vi "Check Loop Error.vi"(6 "Exit on Error? (F)":bool, 7 "Loop Name":string, 8 "Ignore Errors":i32[](array[numeric]), 9 "error to process":errorcluster, 10 "Database":refnum<queue>, 11 "Message Queue":refnum<queue>) -> (2 "Error?":bool, 3 "dup Message Queue":refnum<queue>)   [LabVIEW 2026]
doc: "Check the 'error to process' to see if its code value matches any of the values in the 'Ignore Errors' array. If so, do nothing. If not, send an \"Error\" message containing the error data to the Message Handling Loop for further processing. If the \"Exit on Error?\" input is TRUE, send an \"Exit\" message to the Message Handling Loop instead."
uses:
  Message Queue/Message Cluster.ctl
  controls/Error_Payload.ctl
  Message Queue/Enqueue Message (Single).vi
  Message Queue/Message Queue.lvlib
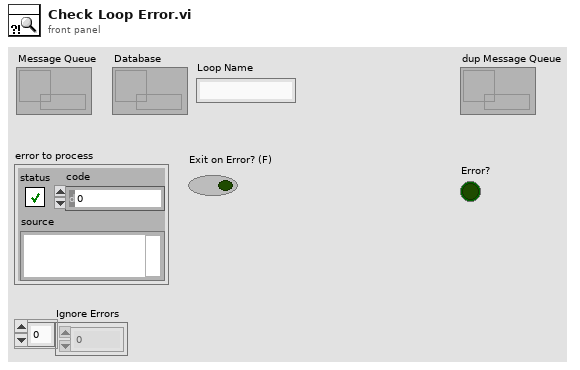
[diagram p1: front panel]
types:
  T1 = typedef "Error_Payload.ctl" = cluster{"status":bool, "error_code":i32, "description":string, "source_loop":string}
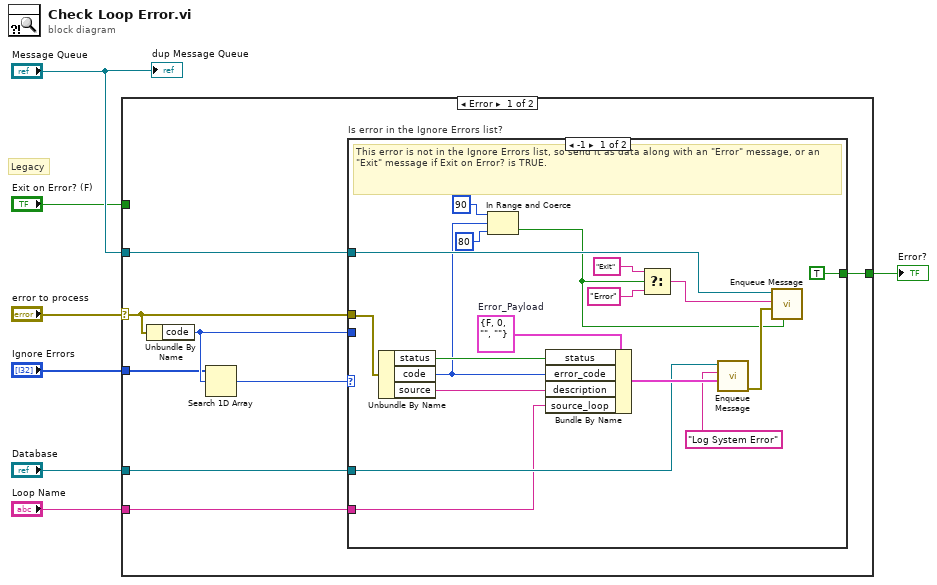
[diagram p0: block diagram]
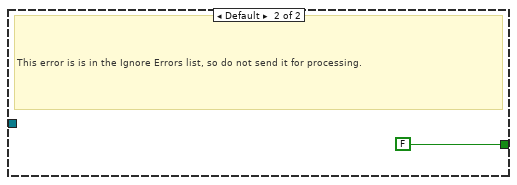
[diagram p2: hidden frame]
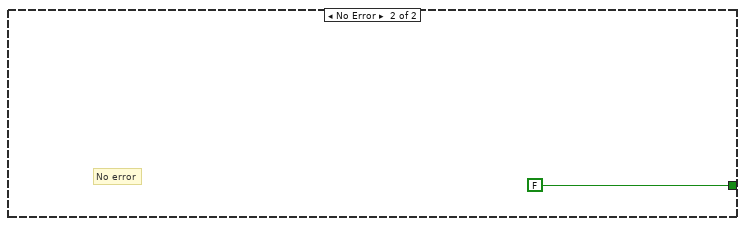
[diagram p3: hidden frame]
diagram:
  # "Legacy"
  n1 = case shown="Error" "error to process" {
    selector: "error to process" -> [w10 _]
    tunnel: "Message Queue" -> [w15 _]
    tunnel: "Ignore Errors" -> [w12 _]
    tunnel: [w11 FALSE] -> w4
    tunnel: "Exit on Error? (F)" -> [_ _]
    tunnel: "Database" -> [w9 _]
    tunnel: "Loop Name" -> [w8 _]
    frame Error {
      n2 = Unbundle By Name(w10) -> ("code"=w13:i32)
      n3 = Search 1D Array(1D array=w12, element=w13) -> (index of element=w14:i32)  [unwired: 1 in]
      n4 = case "Is error in the Ignore Errors list?" shown="-1" w14 {
        tunnel: w10 -> [w25 _]
        tunnel: w15 -> [w33 _]
        tunnel: w13 -> [_ _]
        tunnel: [TRUE FALSE] -> w11
        tunnel: w9 -> [w24 _]
        tunnel: w8 -> [w23 _]
        frame -1 {
          w28 = T1 {"status"=FALSE, "error_code"=0, "description"="", "source_loop"=""}  # Error_Payload
          # "This error is not in the Ignore Errors list, so send it as data along with an \"Error\" message, or an \"Exit\" message if Exit on Error? is TRUE."
          n5 = Unbundle By Name(w25) -> ("status"=w27:bool, "code"=w19:i32, "source"=w20:string)
          n6 = In Range and Coerce(upper limit=90, x=w19, lower limit=80) -> (In Range?=w16:bool)  [unwired: 1 out]
          n7 = Bundle By Name(cluster=w28, "status"=w27, "error_code"=w19, "description"=w20, "source_loop"=w23) -> (w26:T1)
          n8 = Select(t="Exit" ("Message"), s=w16, f="Error" ("Message")) -> (s? t:f=w31:string)
          n9 = call-poly "Enqueue Message.vi"("Message Data"=w26, "Message"="Log System Error", "Message Queue"=w24) -> ("error out"=w21:errorcluster)  [unwired: 7 in, 1 out]
          n10 = call-poly "Enqueue Message.vi"("Priority Message? (F)"=w16, "Message Data"=w21, "Message"=w31, "Message Queue"=w33) -> ()  [unwired: 6 in, 2 out]
        }
        frame Default {
          # "This error is is in the Ignore Errors list, so do not send it for processing."
        }
      }
    }
    frame No Error {
      # "No error"
    }
  }
  "Error?" <- w4
  "dup Message Queue" <- "Message Queue"
